vi "ads.vi"(11 "connection information":path) -> ()   [LabVIEW 2013]
uses:
  <vilib>/addons/database/Connection.llb/DB Tools Open Connec (Path).vi
  <vilib>/addons/database/NI_Database_API.lvlib
panel:
  in  "簇":T1
  in  "注册框":T2
  in  "退出":bool
  in  "登陆":bool
  in  "注册":bool
  out "身份证自动显示":string
  in  "用户姓名":string(combo)
  # "听力测试系统登录界面"
  # "姓名"
  # "身份证号"
  # "姓名"
  # "身份证号码"
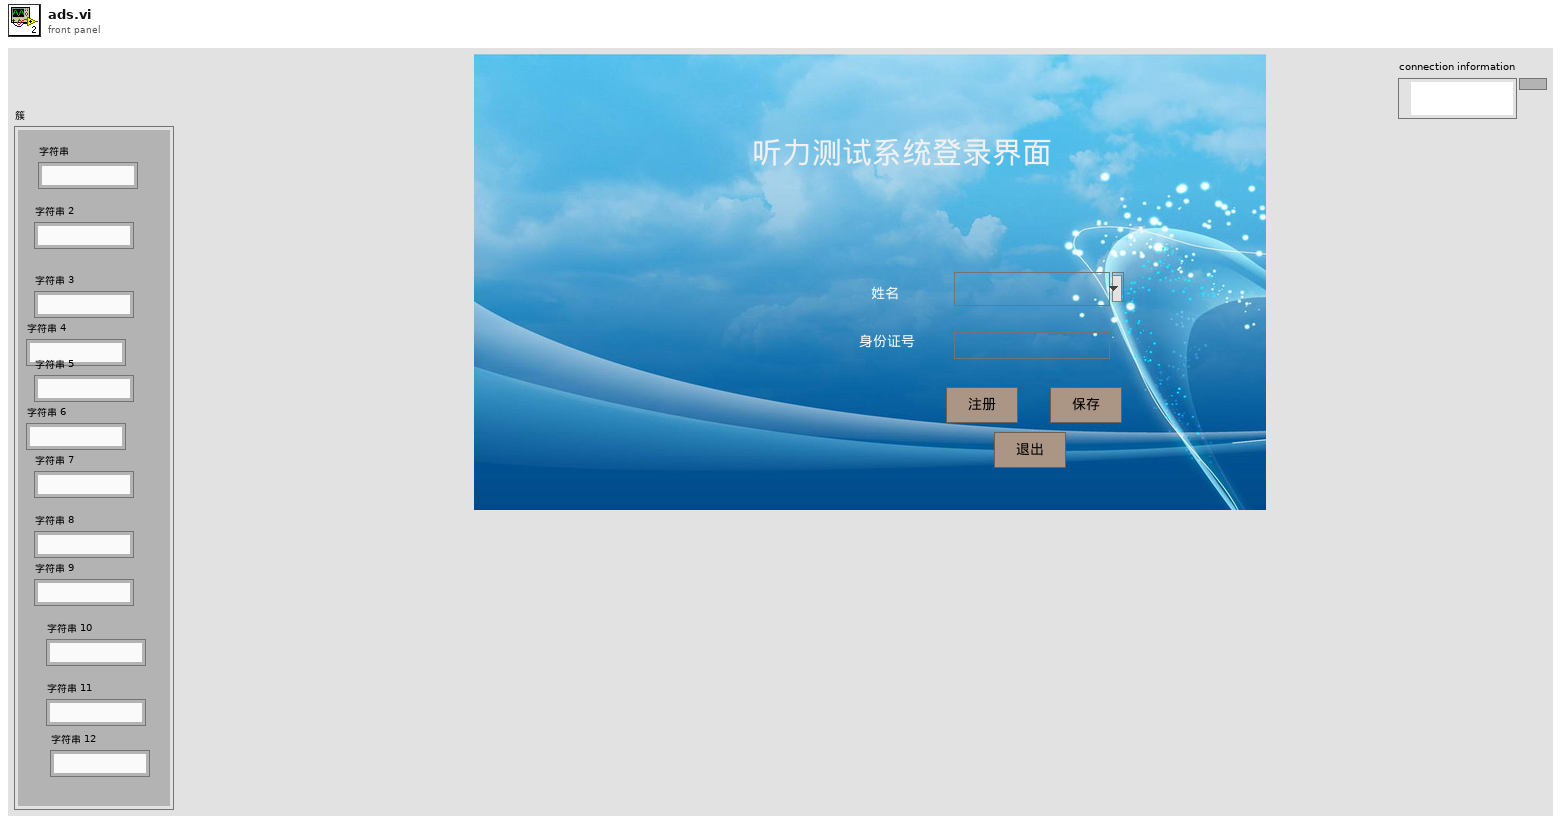
[diagram p1: front panel]
types:
  T1 = cluster{"字符串":string, "字符串 2":string, "字符串 3":string, "字符串 4":string, "字符串 5":string, "字符串 6":string, "字符串 7":string, "字符串 8":string, "字符串 9":string, "字符串 10":string, "字符串 11":string, "字符串 12":string}
  T2 = cluster{"patientname":string, "patientname2":string, "确定注册":bool, "退出":bool, "照相":bool, "性别":enum32{"男", "女"}}
  T3 = typedef "NI_Database_API.lvlib/Conn ObjectReference.ctl" = refnum<k1>
  T4 = cluster{"Value":string, "Value":string, string, string}
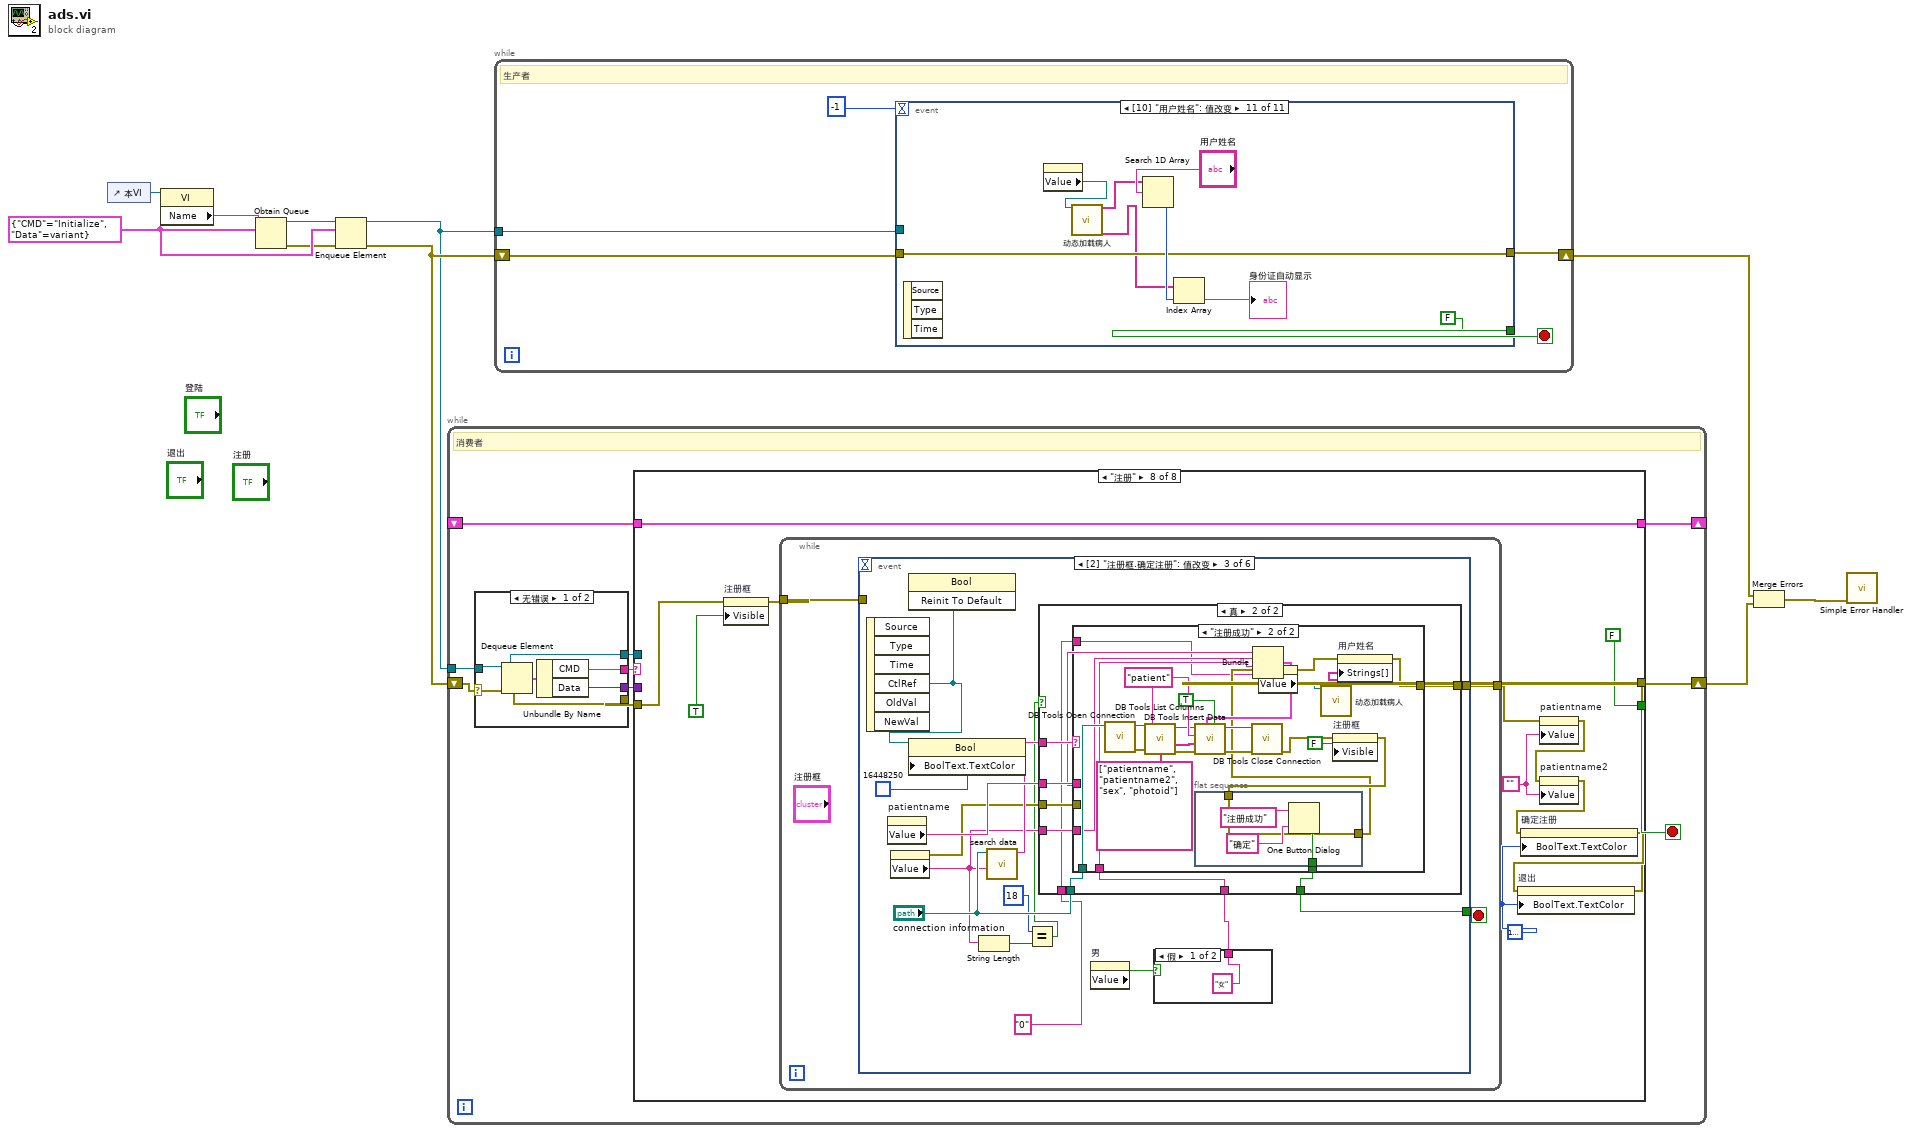
[diagram p0: block diagram]
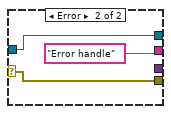
[diagram p2: hidden frame]
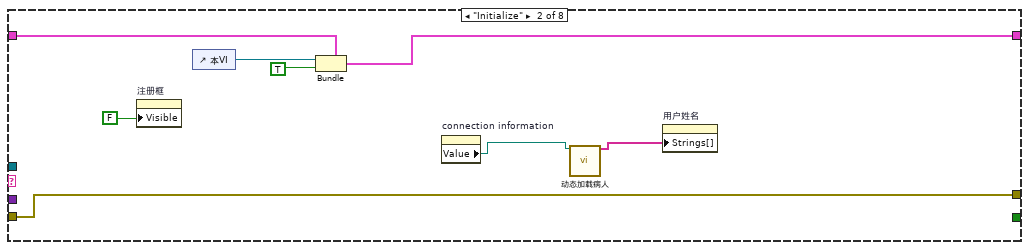
[diagram p4: hidden frame]
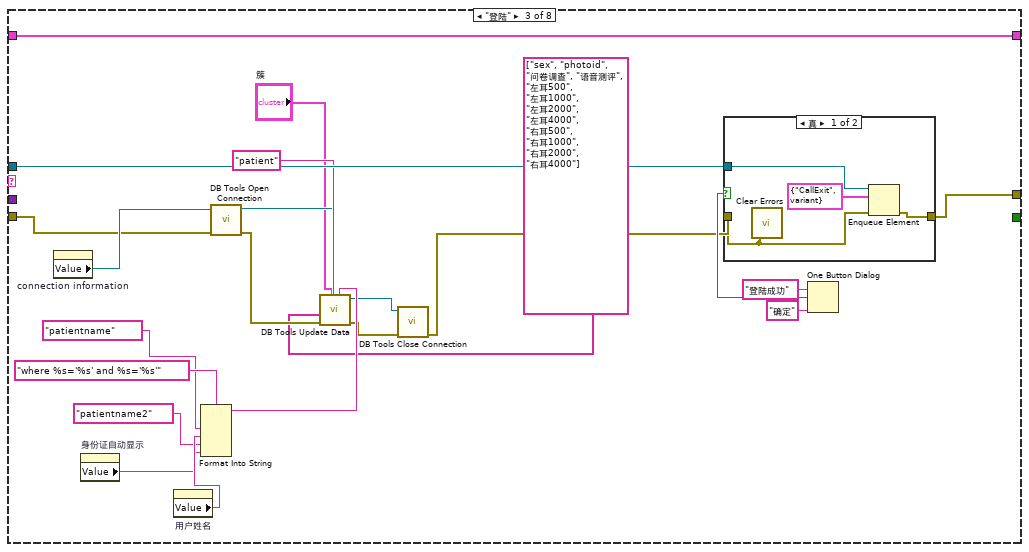
[diagram p5: hidden frame]
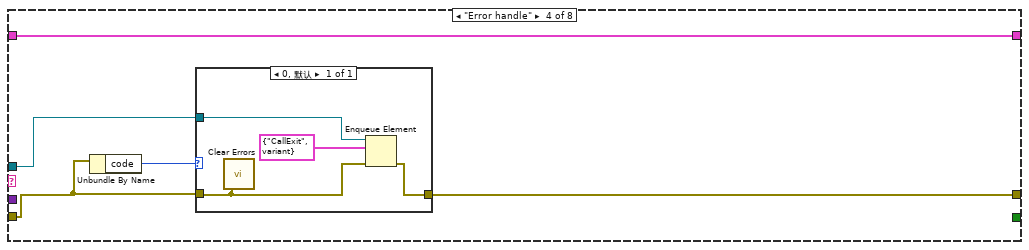
[diagram p7: hidden frame]
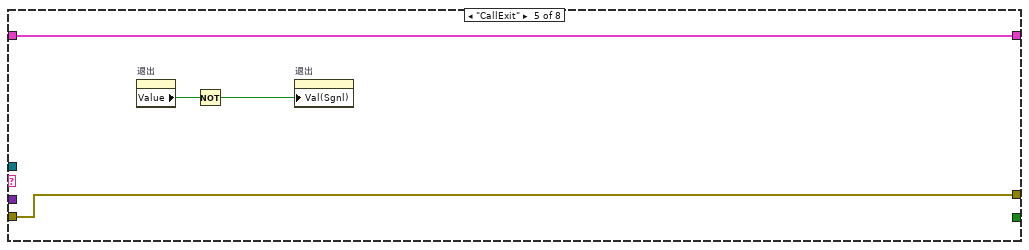
[diagram p8: hidden frame]
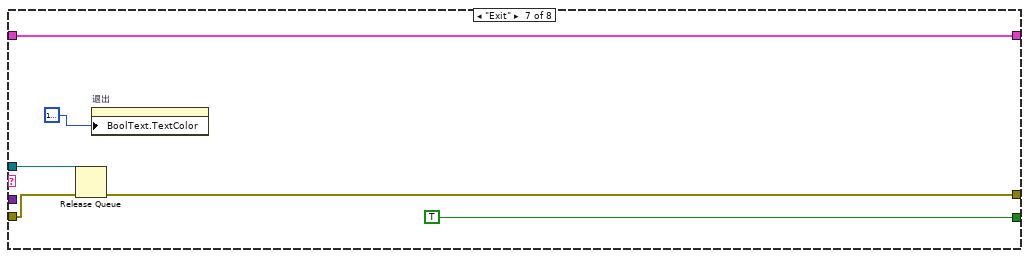
[diagram p10: hidden frame]
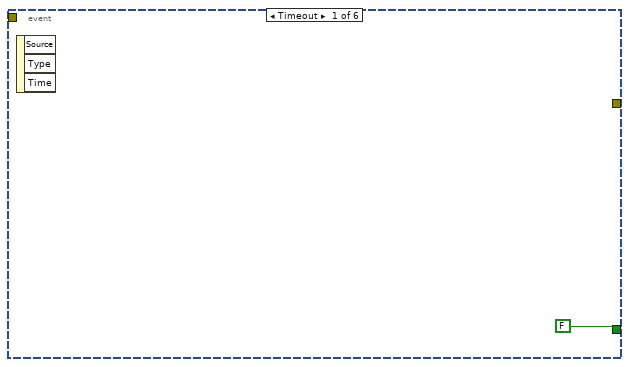
[diagram p11: hidden frame]
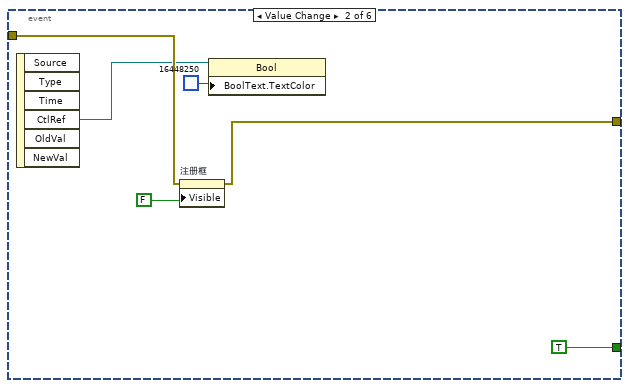
[diagram p12: hidden frame]
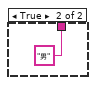
[diagram p13: hidden frame]
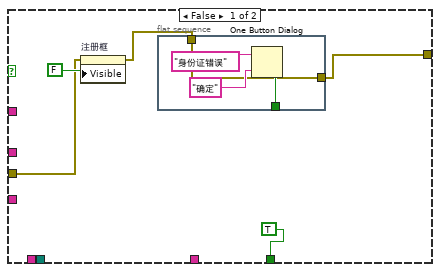
[diagram p14: hidden frame]
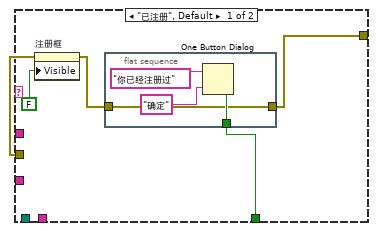
[diagram p15: hidden frame]
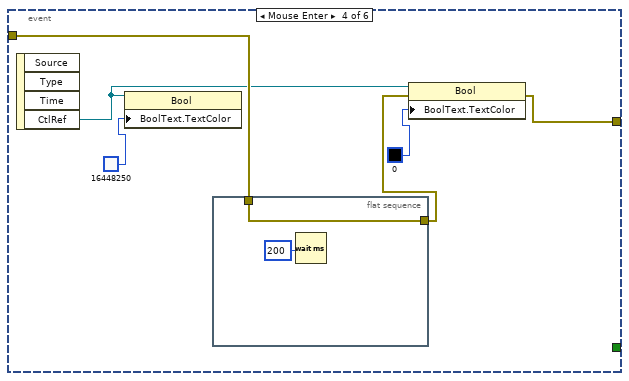
[diagram p16: hidden frame]
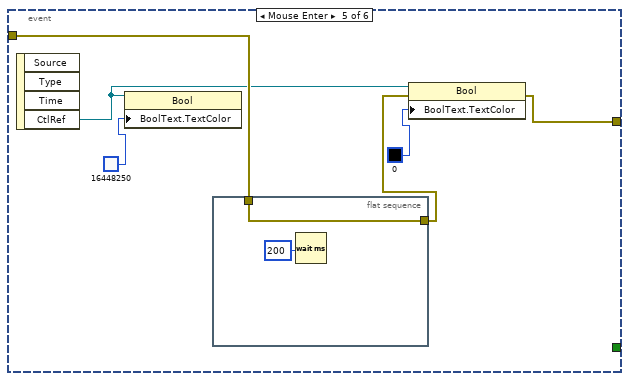
[diagram p17: hidden frame]
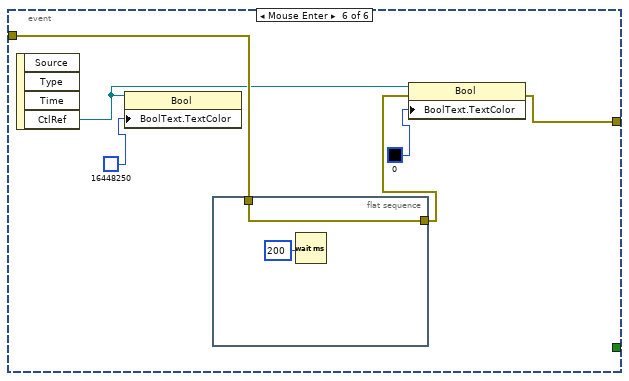
[diagram p18: hidden frame]
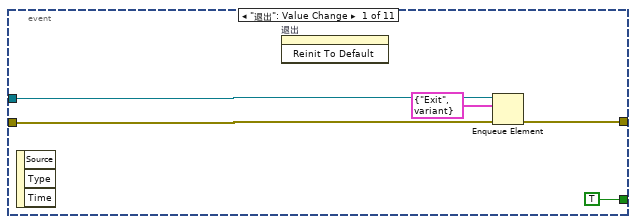
[diagram p19: hidden frame]
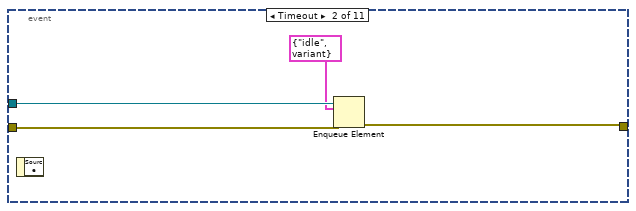
[diagram p20: hidden frame]
diagram:
  w10 = cluster{"CMD":string, "Data":variant} {"CMD"="Initialize", "Data"=variant} ("Q_Data")
  n1 = control-ref of="本VI"() -> (w1:refnum<vi>)
  n2 = property class="VI"(reference=w1) -> ("Name"=w2:string)  [unwired: 1 in, 2 out]
  n3 = Obtain Queue(name (unnamed)=w2, element data type=w10) -> (queue out=w6:refnum<queue>, error out=w8:errorcluster)  [unwired: 3 in, 1 out]
  n4 = Enqueue Element(queue=w6, element=w10, error in (no error)=w8) -> (queue out=w7:refnum<queue>, error out=w9:errorcluster)  [unwired: 1 in, 1 out]
  n5 = while {
    tunnel: w7 -> [w20]
    shift-right: [w15] -> w4
    shift-left: w9 -> [w12]
    shift-right: [w13] -> _
    shift-left: _ -> [w14]
    stop <- w11 stop-if-true
    # "消费者"
    n6 = case shown="无错误" w12 {
      selector: w12 -> [w21 w29]
      tunnel: w20 -> [w27 w30]
      tunnel: [w25 "Error handle"] -> w19
      tunnel: [w24 _] -> w18
      tunnel: [w23 w30] -> w17
      tunnel: [w22 w29] -> w16
      frame No Error {
        n7 = Dequeue Element(queue=w27, error in (no error)=w21) -> (queue out=w23:refnum<queue>, element=w26:cluster{"CMD":string, "Data":variant}, error out=w22:errorcluster)  [unwired: 1 in, 1 out]
        n8 = Unbundle By Name(w26) -> ("CMD"=w25:string, "Data"=w24:variant)
      }
      frame Error {
      }
    }
    n9 = case shown="\"注册\"" w19 {
      tunnel: w18 -> [_ _ _ _ _ _ _ _]
      tunnel: w17 -> [_ _ w59 w69 _ _ w88 _]
      tunnel: w16 -> [w32 w36 w49 w70 w80 w82 w87 w98]
      tunnel: [w32 w36 w58 w68 w80 w82 w86 w89] -> w15
      tunnel: [_ _ _ _ _ _ TRUE FALSE] -> w11
      tunnel: w14 -> [w31 w39 w62 w72 w79 w81 w84 w100]
      tunnel: [w31 w38 w62 w72 w79 w81 w84 w100] -> w13
      frame "idle", Default {
      }
      frame "Initialize" {
        n10 = property on="注册框" class="Clust"("Visible"=FALSE) -> ()  [unwired: 2 in, 2 out]
        n11 = control-ref of="本VI"() -> (w40:refnum<vi>)
        n12 = Bundle(cluster=w39, "本VI"=w40, TRUE) -> (w38:cluster{"本VI":refnum<vi>, bool})
        n13 = property on="connection information" class="Path"() -> ("Value"=w34:path)  [unwired: 2 in, 2 out]
        n14 = call "动态加载病人.vi"("connection information 2"=w34) -> ("姓名"=w33:string[])  [unwired: 15 in, 3 out]
        n15 = property on="用户姓名" class="CmbBox"("Strings[]"=w33) -> ()  [unwired: 2 in, 2 out]
      }
      frame "登陆" {
        n16 = property on="connection information" class="Path"() -> ("Value"=w56:path)  [unwired: 2 in, 2 out]
        n17 = property on="身份证自动显示" class="Str"() -> ("Value"=w43:string)  [unwired: 2 in, 2 out]
        n18 = property on="用户姓名" class="CmbBox"() -> ("Value"=w45:string)  [unwired: 2 in, 2 out]
        n19 = Format Into String(format string="where %s='%s' and %s='%s'" ("condition"), "patientname", w45, "patientname2", w43) -> (resulting string=w52:string)  [unwired: 2 in, 1 out]
        n20 = call-poly <vilib>:"DB Tools Open Connection.vi"("error in (no error)"=w49, "connection information"=w56) -> ("error out"=w48:errorcluster, "connection reference"=w54:T3)  [unwired: 6 in]
        n21 = call <vilib>:"DB Tools Update Data.vi"("condition"=w52, "data"="簇", "error in (no error)"=w48, "columns"=string[] ["sex", "photoid", "问卷调查", "语音测评", "左耳500", "左耳1000", "左耳2000", "左耳4000", "右耳500", "右耳1000", "右耳2000", "右耳4000"], "table"="patient", "connection reference"=w54) -> ("error out"=w50:errorcluster, "connection reference out"=w51:T3)  [unwired: 4 in]
        n22 = call <vilib>:"DB Tools Close Connection.vi"("error in (no error)"=w50, "connection reference"=w51) -> ("error out"=w47:errorcluster)  [unwired: 5 in]
        n23 = One Button Dialog(message="登陆成功" ("消息"), button name ("OK")="确定" ("按钮名称（“确定”）")) -> (true=w57:bool)
        n24 = case shown="真" w57 {
          tunnel: w47 -> [w64 w67]
          tunnel: w59 -> [w65 _]
          tunnel: [w63 w67] -> w58
          frame True {
            n25 = call <vilib>:"Clear Errors.vi"("error in (no error)"=w64) -> ()  [unwired: 6 in, 1 out]
            n26 = Enqueue Element(queue=w65, element=cluster{"CMD":string, "Data":variant} {"CMD"="CallExit", "Data"=variant} ("元素"), error in (no error)=w64) -> (error out=w63:errorcluster)  [unwired: 1 in, 2 out]
          }
          frame False {
          }
        }
      }
      frame "Error handle" {
        n27 = Unbundle By Name(w70) -> ("code"=w71:i32)
        n28 = case shown="0, 默认" w71 {
          tunnel: w70 -> [w74]
          tunnel: w69 -> [w75]
          tunnel: [w73] -> w68
          frame 0, Default {
            n29 = call <vilib>:"Clear Errors.vi"("error in (no error)"=w74) -> ()  [unwired: 6 in, 1 out]
            n30 = Enqueue Element(queue=w75, element=cluster{"CMD":string, "Data":variant} {"CMD"="CallExit", "Data"=variant} ("元素"), error in (no error)=w74) -> (error out=w73:errorcluster)  [unwired: 1 in, 2 out]
          }
        }
      }
      frame "CallExit" {
        n31 = property on="退出" class="Bool (严格)"() -> ("Value"=w78:bool)  [unwired: 2 in, 2 out]
        n32 = Not(x=w78) -> (.not. x?=w77:bool)
        n33 = property on="退出" class="Bool (严格)"("Val(Sgnl)"=w77) -> ()  [unwired: 2 in, 2 out]
      }
      frame "--------user--------" {
      }
      frame "Exit" {
        n34 = Release Queue(queue=w88, error in (no error)=w87) -> (error out=w86:errorcluster)  [unwired: 1 in, 2 out]
        n35 = property on="退出" class="Bool (严格)"("BoolText.TextColor"=u32 16777222 ("颜色盒")) -> ()  [unwired: 2 in, 2 out]
      }
      frame "注册" {
        w92 = u32 16777228 ("颜色盒")
        w93 = ""
        n36 = property on="注册框" class="Clust"(error in=w98, "Visible"=TRUE) -> (error out=w97:errorcluster)  [unwired: 1 in, 1 out]
        n37 = while {
          tunnel: [w102] -> w94
          tunnel: w97 -> [w101]
          stop <- w103 stop-if-true
          n38 = event shown="[2] \"注册框.确定注册\": 值改变" {
            selector: _ -> [_ _ _ _ _ _]
            dyn-events: _ -> [_ _ _ _ _ _]
            timeout: _ -> [_ _ _ _ _ _]
            tunnel: [FALSE TRUE w121 _ _ _] -> w103
            tunnel: [_ w107 w125 w183 w191 w199] -> w102
            tunnel: w101 -> [_ w108 _ w187 w195 w203]
            event Timeout {
              n39 = event-data() -> ()  [unwired: 1 in, 3 out]
            }
            event "注册框.退出": Value Change {
              n40 = event-data() -> ("CtlRef"=w105:refnum<vi>)  [unwired: 1 in, 5 out]
              n41 = property on="注册框" class="Clust"(error in=w108, "Visible"=FALSE) -> (error out=w107:errorcluster)  [unwired: 1 in, 1 out]
              n42 = property class="Bool"(reference=w105, "BoolText.TextColor"=u32 16448250 ("颜色盒")) -> ()  [unwired: 1 in, 2 out]
            }
            event "注册框.确定注册": Value Change {
              n43 = event-data() -> ("CtlRef"=w115:refnum<vi>)  [unwired: 1 in, 5 out]
              n44 = property on="patientname" class="Str"() -> ("Value"=w124:string)  [unwired: 2 in, 2 out]
              n45 = property on="patientname2" class="Str"() -> (error out=w120:errorcluster, "Value"=w119:string)  [unwired: 2 in, 1 out]
              n46 = invoke class="Bool" method="Reinit To Default"(reference=w115) -> ()  [unwired: 2 in, 3 out]
              n47 = property class="Bool"(reference=w115, "BoolText.TextColor"=u32 16448250 ("颜色盒")) -> ()  [unwired: 1 in, 2 out]
              n48 = String Length(string=w119) -> (length=w117:i32)
              n49 = call "search data.vi"("y"=w119, "connection information"="connection information") -> ("字符串"=w122:string)  [unwired: 9 in]
              n50 = Equal?(x=18, y=w117) -> (x = y?=w116:bool)
              n51 = property on="男" class="Bool (严格)"() -> ("Value"=w113:bool)  [unwired: 2 in, 2 out]
              n52 = case shown="假" w113 {
                tunnel: ["女" "男"] -> w112
                frame False {
                }
                frame True {
                }
              }
              n53 = case shown="真" w116 {
                tunnel: [w128 w145] -> w125
                tunnel: w124 -> [_ w144]
                tunnel: "connection information" -> [_ w143]
                tunnel: w122 -> [_ w142]
                tunnel: [TRUE w141] -> w121
                tunnel: w120 -> [w130 w140]
                tunnel: w119 -> [_ w139]
                tunnel: w112 -> [_ w138]
                tunnel: "0" -> [_ w137]
                frame False {
                  n54 = property on="注册框" class="Clust"(error in=w130, "Visible"=FALSE) -> (error out=w129:errorcluster)  [unwired: 1 in, 1 out]
                  n55 = flat-sequence {
                    tunnel: w129 -> [w133]
                    tunnel: [w134] -> _
                    tunnel: [w133] -> w128
                    frame #0 {
                      n56 = One Button Dialog(message="身份证错误" ("Message"), button name ("OK")="确定") -> (true=w134:bool)
                    }
                  }
                }
                frame True {
                  n57 = case shown="\"注册成功\"" w142 {
                    tunnel: [w146 w160] -> w145
                    tunnel: w144 -> [_ w169]
                    tunnel: w143 -> [_ w168]
                    tunnel: [w150 w167] -> w141
                    tunnel: w140 -> [w148 _]
                    tunnel: w139 -> [_ w165]
                    tunnel: w138 -> [_ w158]
                    tunnel: w137 -> [_ w157]
                    frame "已注册", Default {
                      n58 = property on="注册框" class="Clust"(error in=w148, "Visible"=FALSE) -> (error out=w147:errorcluster)  [unwired: 1 in, 1 out]
                      n59 = flat-sequence {
                        tunnel: [w152] -> w150
                        tunnel: w147 -> [w151]
                        tunnel: [w151] -> w146
                        frame #0 {
                          n60 = One Button Dialog(message="你已经注册过" ("Message"), button name ("OK")="确定") -> (true=w152:bool)
                        }
                      }
                    }
                    frame "注册成功" {
                      w178 = "patient" ("table")
                      n61 = call-poly <vilib>:"DB Tools Open Connection.vi"("connection information"=w168) -> ("error out"=w174:errorcluster, "connection reference"=w164:T3)  [unwired: 7 in]
                      n62 = call <vilib>:"DB Tools List Columns.vi"("error in (no error)"=w174, "table"=w178, "connection reference"=w164) -> ("error out"=w177:errorcluster, "connection reference out"=w175:T3)  [unwired: 1 in, 2 out]
                      n63 = flat-sequence {
                        tunnel: w163 -> [w179]
                        tunnel: [w180] -> w167
                        tunnel: [w179] -> w162
                        frame #0 {
                          n64 = One Button Dialog(message="注册成功" ("Message"), button name ("OK")="确定") -> (true=w180:bool)
                        }
                      }
                      n65 = Bundle("Value"=w169, "Value"=w165, w158, w157) -> (w170:T4)  [unwired: 1 in]
                      n66 = call <vilib>:"DB Tools Insert Data.vi"("create table? (F)"=TRUE, "data"=w170, "error in (no error)"=w177, "columns"=string[] ["patientname", "patientname2", "sex", "photoid"], "table"=w178, "connection reference"=w175) -> ("error out"=w176:errorcluster, "connection reference out"=w166:T3)  [unwired: 4 in]
                      n67 = call <vilib>:"DB Tools Close Connection.vi"("error in (no error)"=w176, "connection reference"=w166) -> ("error out"=w173:errorcluster)  [unwired: 5 in]
                      n68 = property on="connection information" class="Path"(error in=w162) -> (error out=w161:errorcluster, "Value"=w156:path)  [unwired: 1 in, 1 out]
                      n69 = call "动态加载病人.vi"("connection information 2"=w156) -> ("姓名"=w155:string[])  [unwired: 15 in, 3 out]
                      n70 = property on="注册框" class="Clust"(error in=w173, "Visible"=FALSE) -> (error out=w163:errorcluster)  [unwired: 1 in, 1 out]
                      n71 = property on="用户姓名" class="CmbBox"(error in=w161, "Strings[]"=w155) -> (error out=w160:errorcluster)  [unwired: 1 in, 1 out]
                    }
                  }
                }
              }
            }
            event "注册框.确定注册": Mouse Enter {
              n72 = event-data() -> ("CtlRef"=w185:refnum<vi>)  [unwired: 1 in, 3 out]
              n73 = property class="Bool"(reference=w185, "BoolText.TextColor"=u32 16448250 ("颜色盒")) -> ()  [unwired: 1 in, 2 out]
              n74 = flat-sequence {
                tunnel: w187 -> [w189]
                tunnel: [w189] -> w184
                frame #0 {
                  n75 = Wait (ms)(milliseconds to wait=200) -> ()  [unwired: 1 out]
                }
              }
              n76 = property class="Bool"(reference=w185, error in=w184, "BoolText.TextColor"=u32 0 ("颜色盒")) -> (error out=w183:errorcluster)  [unwired: 1 out]
            }
            event "注册框.退出": Mouse Enter {
              n77 = event-data() -> ("CtlRef"=w193:refnum<vi>)  [unwired: 1 in, 3 out]
              n78 = property class="Bool"(reference=w193, "BoolText.TextColor"=u32 16448250 ("颜色盒")) -> ()  [unwired: 1 in, 2 out]
              n79 = flat-sequence {
                tunnel: w195 -> [w197]
                tunnel: [w197] -> w192
                frame #0 {
                  n80 = Wait (ms)(milliseconds to wait=200) -> ()  [unwired: 1 out]
                }
              }
              n81 = property class="Bool"(reference=w193, error in=w192, "BoolText.TextColor"=u32 0 ("颜色盒")) -> (error out=w191:errorcluster)  [unwired: 1 out]
            }
            event "注册框.照相": Mouse Enter {
              n82 = event-data() -> ("CtlRef"=w201:refnum<vi>)  [unwired: 1 in, 3 out]
              n83 = property class="Bool"(reference=w201, "BoolText.TextColor"=u32 16448250 ("颜色盒")) -> ()  [unwired: 1 in, 2 out]
              n84 = flat-sequence {
                tunnel: w203 -> [w205]
                tunnel: [w205] -> w200
                frame #0 {
                  n85 = Wait (ms)(milliseconds to wait=200) -> ()  [unwired: 1 out]
                }
              }
              n86 = property class="Bool"(reference=w201, error in=w200, "BoolText.TextColor"=u32 0 ("颜色盒")) -> (error out=w199:errorcluster)  [unwired: 1 out]
            }
          }
        }
        n87 = property on="patientname" class="Str"(error in=w94, "Value"=w93) -> (error out=w95:errorcluster)  [unwired: 1 in, 1 out]
        n88 = property on="patientname2" class="Str"(error in=w95, "Value"=w93) -> (error out=w91:errorcluster)  [unwired: 1 in, 1 out]
        n89 = property on="确定注册" class="Bool"(error in=w91, "BoolText.TextColor"=w92) -> (error out=w90:errorcluster)  [unwired: 1 in, 1 out]
        n90 = property on="退出" class="Bool"(error in=w90, "BoolText.TextColor"=w92) -> (error out=w89:errorcluster)  [unwired: 1 in, 1 out]
      }
    }
  }
  n91 = while {
    shift-right: [w210] -> w3
    shift-left: w9 -> [w207]
    tunnel: w7 -> [w208]
    stop <- w209 stop-if-true
    # "生产者"
    n92 = event shown="[10] \"用户姓名\": 值改变" {
      selector: _ -> [_ _ _ _ _ _ _ _ _ _ _]
      dyn-events: _ -> [_ _ _ _ _ _ _ _ _ _ _]
      timeout: -1 -> [_ _ _ _ _ _ _ _ _ _ _]
      tunnel: w208 -> [w212 w220 w224 w227 _ _ _ _ _ _ _]
      tunnel: w207 -> [w214 w219 w223 w226 _ _ _ _ _ _ w238]
      tunnel: [w213 w217 w221 w225 _ _ _ _ _ _ w238] -> w210
      tunnel: [TRUE _ _ _ _ _ _ _ _ _ FALSE] -> w209
      event "退出": Value Change {
        n93 = event-data() -> ()  [unwired: 1 in, 3 out]
        n94 = invoke on="退出" class="Bool (严格)" method="Reinit To Default"() -> ()  [unwired: 3 in, 3 out]
        n95 = Enqueue Element(queue=w212, element=cluster{"CMD":string, "Data":variant} {"CMD"="Exit", "Data"=variant} ("元素"), error in (no error)=w214) -> (error out=w213:errorcluster)  [unwired: 1 in, 2 out]
      }
      event Timeout {
        n96 = event-data() -> ()  [unwired: 1 in, 1 out]
        n97 = Enqueue Element(queue=w220, element=cluster{"CMD":string, "Data":variant} {"CMD"="idle", "Data"=variant} ("元素"), error in (no error)=w219) -> (error out=w217:errorcluster)  [unwired: 1 in, 2 out]
      }
      event "注册": Value Change {
        n98 = event-data() -> ()  [unwired: 1 in, 3 out]
        n99 = Enqueue Element(queue=w224, element=cluster{"CMD":string, "Data":variant} {"CMD"="注册", "Data"=variant} ("元素"), error in (no error)=w223) -> (error out=w221:errorcluster)  [unwired: 1 in, 2 out]
        n100 = invoke on="注册" class="Bool" method="Reinit To Default"() -> ()  [unwired: 3 in, 3 out]
      }
      event "登陆": Value Change {
        n101 = event-data() -> ()  [unwired: 1 in, 3 out]
        n102 = invoke on="登陆" class="Bool" method="Reinit To Default"() -> ()  [unwired: 3 in, 3 out]
        n103 = Enqueue Element(queue=w227, element=cluster{"CMD":string, "Data":variant} {"CMD"="登陆", "Data"=variant} ("元素"), error in (no error)=w226) -> (error out=w225:errorcluster)  [unwired: 1 in, 2 out]
      }
      event "注册": Mouse Enter {
        n104 = event-data() -> ()  [unwired: 1 in, 3 out]
        n105 = property on="注册" class="Bool"("BoolText.TextColor"=u32 16448250 ("颜色盒")) -> ()  [unwired: 2 in, 2 out]
      }
      event "登陆": Mouse Enter {
        n106 = event-data() -> ()  [unwired: 1 in, 3 out]
        n107 = property on="登陆" class="Bool"("BoolText.TextColor"=u32 16448250 ("颜色盒")) -> ()  [unwired: 2 in, 2 out]
      }
      event "退出": Mouse Enter {
        n108 = event-data() -> ()  [unwired: 1 in, 3 out]
        n109 = property on="退出" class="Bool (严格)"("BoolText.TextColor"=u32 16448250 ("颜色盒")) -> ()  [unwired: 2 in, 2 out]
      }
      event "注册": Mouse Leave {
        n110 = event-data() -> ()  [unwired: 1 in, 3 out]
        n111 = property on="注册" class="Bool"("BoolText.TextColor"=u32 16777222 ("颜色盒")) -> ()  [unwired: 2 in, 2 out]
      }
      event "登陆": Mouse Leave {
        n112 = event-data() -> ()  [unwired: 1 in, 3 out]
        n113 = property on="登陆" class="Bool"("BoolText.TextColor"=u32 16777222 ("颜色盒")) -> ()  [unwired: 2 in, 2 out]
      }
      event "退出": Mouse Leave {
        n114 = event-data() -> ()  [unwired: 1 in, 3 out]
        n115 = property on="退出" class="Bool (严格)"("BoolText.TextColor"=u32 16777222 ("颜色盒")) -> ()  [unwired: 2 in, 2 out]
      }
      event "用户姓名": Value Change {
        n116 = event-data() -> ()  [unwired: 1 in, 3 out]
        n117 = property on="connection information" class="Path"() -> ("Value"=w237:path)  [unwired: 2 in, 2 out]
        n118 = call "动态加载病人.vi"("connection information 2"=w237) -> ("姓名"=w236:string[], "身份证"=w235:string[])  [unwired: 15 in, 2 out]
        n119 = Search 1D Array(1D array=w236, element="用户姓名") -> (index of element=w242:i32)  [unwired: 1 in]
        n120 = Index Array(array=w235, index=w242) -> (element=→"身份证自动显示":string)
      }
    }
  }
  n121 = Merge Errors(w3, w4) -> (w5:errorcluster)
  n122 = call <vilib>:"Simple Error Handler.vi"("error in (no error)"=w5) -> ()  [unwired: 4 in, 5 out]
